vi "Close Client.vi"(8 "error in (no error)":errorcluster, 11 "Client in":refnum<class "Client.lvclass">) -> (0 "error out":errorcluster)   [LabVIEW 2020, in "Client.lvlib"]
doc: "Close the PVAccess client."
uses:
  Client.lvlib
  Client/Client.lvclass
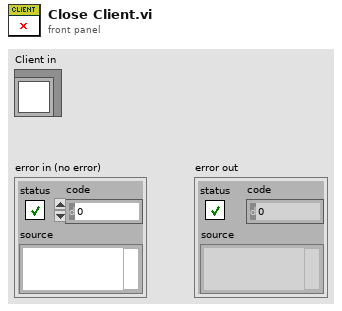
[diagram p1: front panel]
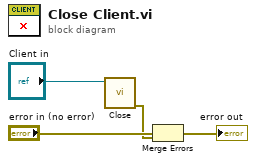
[diagram p0: block diagram]
diagram:
  n1 = call "Close.vi"("Client in"="Client in") -> ("error out"=w2:errorcluster)  [unwired: 9 in, 1 out]
  n2 = Merge Errors("error in (no error)", w2) -> (→"error out":errorcluster)
